vi "LVClass_ModalCoef SetCoefsValues.vi"(0 "ModalCoef in":refnum<class "ModalCoef.lvclass">, 5 "coef":sgl[](array[numeric]), 7 "index":u32[](array[numeric]), 11 "error in (no error)":errorcluster) -> (4 "ModalCoef out":refnum<class "ModalCoef.lvclass">, 8 "index":u32[](array[numeric]), 15 "error out":errorcluster)   [LabVIEW 2020, in "ModalCoef.lvclass"]
doc: "Set polynomial coefficients informations and values.\n\n--------------------------------------------------------------------------------\n\n<B>TypePhaseIn </B> : TypePhase phase mode reconstruction.\n<B>TypePhaseOut </B> : TypePhase phase mode reconstruction.\n<B>modalCoef </B> : ModalCoef object.\n<B>coef </B> : Array of modal coefficient values.\n<B>index </B> : Array of modal coefficient indices.\n<B>size </B> : Size of the coefficient array.\n<B>pupil </B> : pupil object.\n<B>ErrorIn </B> : Error\n<B>ErrorOut </B> : Error\n\n--------------------------------------------------------------------------------"
uses:
  ModalCoef.lvclass
  ModalCoef.lvclass/ModalCoef.ctl
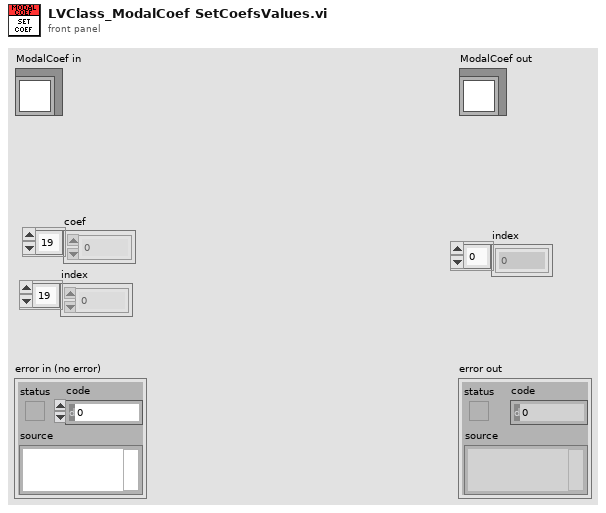
[diagram p1: front panel]
types:
  T1 = typedef "ClassID.ctl" = i64
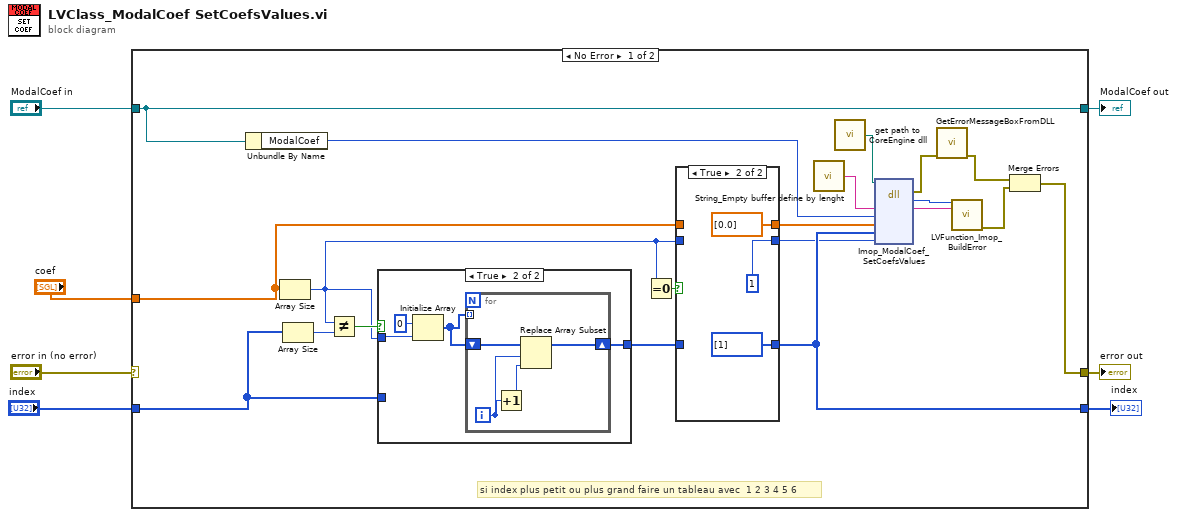
[diagram p0: block diagram]
diagram:
  n1 = case shown="No Error" "error in (no error)" {
    selector: "error in (no error)" -> [_ w45]
    tunnel: [w16 w45] -> w6
    tunnel: [w21 w44] -> w4
    tunnel: "ModalCoef in" -> [w21 w44]
    tunnel: [w10 w43] -> w3
    tunnel: "index" -> [w15 w43]
    tunnel: "coef" -> [w12 _]
    frame No Error {
      # "si index plus petit ou plus grand faire un tableau avec  1 2 3 4 5 6"
      n2 = Unbundle By Name(w21) -> ("ModalCoef"=w22:T1)
      n3 = Array Size(array=w12) -> (size(s)=w8:i32)
      n4 = Array Size(array=w15) -> (size(s)=w20:i32)
      n5 = Not Equal?(x=w8, y=w20) -> (x != y?=w19:bool)
      n6 = case shown="True" w19 {
        tunnel: w8 -> [_ w36]
        tunnel: w15 -> [w34 _]
        tunnel: [w34 w35] -> w14
        frame False {
        }
        frame True {
          n7 = Initialize Array(u32 0, w36) -> (w37:u32[])
          n8 = for {
            shift-right: [w39] -> w35
            shift-left: w37 -> [w40]
            tunnel: w37 -> [_] mode=indexing
            i -> [w41]
            n9 = Increment(x=w41) -> (x+1=w42:i32)
            n10 = Replace Array Subset(array=w40, new element=w42, index=w41) -> (w39:u32[])
          }
        }
      }
      n11 = Equal To 0?(x=w8) -> (x = 0?=w13:bool)
      n12 = case shown="True" w13 {
        tunnel: w14 -> [w29 _]
        tunnel: w12 -> [w30 _]
        tunnel: [w30 sgl[] [0.0] ("coef")] -> w11
        tunnel: [w29 u32[] [1] ("index")] -> w10
        tunnel: [w28 u32 1] -> w9
        tunnel: w8 -> [w28 _]
        frame False {
        }
        frame True {
        }
      }
      n13 = call "String_Empty buffer define by lenght.vi"() -> ("Empty buffer"=w27:string)  [unwired: 1 in]
      n14 = call "get path to CoreEngine dll.vi"() -> ("path to wavekit library"=w24:path)  [unwired: 14 in, 1 out]
      n15 = dll-call lib="D:/2_trunk/Soft_haso/ImOpCoreEngine4_LV2011/DLLs/ImopEngine4_vc100.dll" fn="Imop_ModalCoef_SetCoefsValues"(path in=w24, "message"=w27, "ModalCoefs"=w22, "coef"=w11, "index"=w10, "size"=w9) -> (error out=w23:errorcluster, "return type"=w25:i32, "message"=w26:string)  [unwired: 6 in, 1 out]
      n16 = call "GetErrorMessageBoxFromDLL.vi"("error IN"=w23) -> ("error OUT"=w18:errorcluster)  [unwired: 10 in]
      n17 = call "LVFunction_Imop_BuildError.vi"("code"=w25, "String to Prepend to source (\"\")"=w26) -> ("error out"=w17:errorcluster)  [unwired: 13 in]
      n18 = Merge Errors(w18, w17) -> (w16:errorcluster)
    }
    frame Error {
    }
  }
  "error out" <- w6
  "ModalCoef out" <- w4
  "index" <- w3
